vi "Update ceeserver applications.vi"(2 "Source directory":path=path "C:/Users/mw24/Documents/LabVIEW Data/builds") -> (0 "Current file":string)   [LabVIEW 2010]
panel:
  out "uploaded files":string[](array[string])
  out "move to path":path
  out "exe":string[](array[string])
  out "htm":string[](array[string])
  in  "Destination directory":path=path "\\\\ceeserver.cee.cornell.edu\\mw24/Software/Runtime2010"
  out "Current destination":string
  out "file names":string[](array[string])
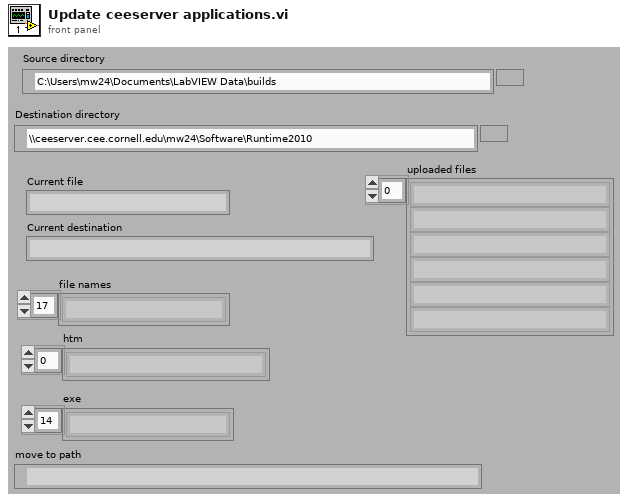
[diagram p1: front panel]
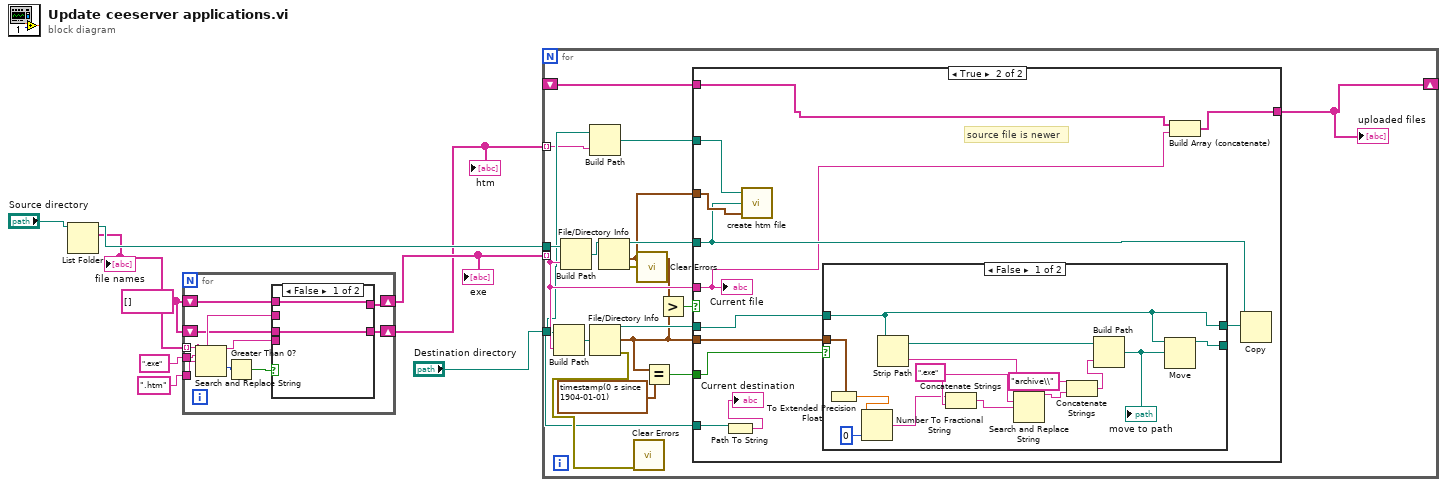
[diagram p0: block diagram]
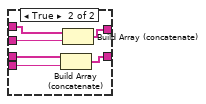
[diagram p2: hidden frame]
diagram:
  w3 = string[] []
  n1 = List Folder(path="Source directory") -> (path out=w8:path, filenames=w6:string[])  [unwired: 3 in, 2 out]
  "file names" <- w6
  n2 = for {
    tunnel: w6 -> [w15] mode=indexing
    tunnel: ".exe" ("search string") -> [w18]
    shift-right: [w17] -> w4
    shift-left: w3 -> [w14]
    shift-right: [w13] -> w2
    shift-left: w3 -> [w11]
    tunnel: ".htm" ("search string") -> [w10]
    n3 = Search and Replace String(input string=w15, search string=w18, replace string=w10) -> (result string=w12:string, offset past replacement=w19:i32)  [unwired: 5 in, 2 out]
    n4 = Greater Than 0?(x=w19) -> (x > 0?=w16:bool)
    n5 = case shown="False" w16 {
      tunnel: [w21 w27] -> w17
      tunnel: w15 -> [_ w26]
      tunnel: w14 -> [w21 w25]
      tunnel: [w20 w24] -> w13
      tunnel: w12 -> [_ w23]
      tunnel: w11 -> [w20 w22]
      frame False {
      }
      frame True {
        n6 = Build Array (concatenate)(w22, w23) -> (w24:string[])
        n7 = Build Array (concatenate)(w25, w26) -> (w27:string[])
      }
    }
  }
  "htm" <- w2
  "exe" <- w4
  n8 = for {
    tunnel: w4 -> [w39] mode=indexing
    tunnel: w8 -> [w45]
    tunnel: "Destination directory" -> [w33]
    tunnel: w2 -> [w32] mode=indexing
    shift-right: [w28] -> _
    shift-left: _ -> [w29]
    n9 = Build Path(base path=w33, name or relative path=w39) -> (appended path=w43:path)
    n10 = Build Path(base path=w45, name or relative path=w39) -> (appended path=w44:path)
    n11 = Build Path(base path=w33, name or relative path=w32) -> (appended path=w31:path)
    n12 = File/Directory Info(path=w43) -> (path out=w41:path, last mod=w30:timestamp, error out=w35:errorcluster)  [unwired: 1 in, 4 out]
    n13 = File/Directory Info(path=w44) -> (path out=w40:path, last mod=w34:timestamp, error out=w38:errorcluster)  [unwired: 1 in, 4 out]
    n14 = call <vilib>:"Clear Errors.vi"("error in (no error)"=w35) -> ()  [unwired: 6 in, 1 out]
    n15 = call <vilib>:"Clear Errors.vi"("error in (no error)"=w38) -> ()  [unwired: 6 in, 1 out]
    n16 = Equal?(x=w30, y=timestamp(0 s since 1904-01-01) ("last mod")) -> (x = y?=w36:bool)
    n17 = Greater?(x=w34, y=w30) -> (0:w42:bool)
    n18 = case shown="True" w42 {
      tunnel: w40 -> [_ w51]
      tunnel: w41 -> [_ w57]
      tunnel: w39 -> [_ w47]
      tunnel: w33 -> [_ w55]
      tunnel: w36 -> [_ w56]
      tunnel: w34 -> [_ w54]
      tunnel: w31 -> [_ w52]
      tunnel: w30 -> [_ w53]
      tunnel: [w46 w48] -> w28
      tunnel: w29 -> [w46 w49]
      frame False {
        # "source file is same age as file on ceeserver"
      }
      frame True {
        # "source file is newer"
        n19 = Path To String(path=w55) -> (string=→"Current destination":string)
        n20 = call "create htm file.vi"("last mod"=w54, "Source path"=w51, "Destination path"=w52) -> ()  [unwired: 2 in]
        n21 = case shown="False" w56 {
          tunnel: w57 -> [w72 w73]
          tunnel: [w72 w73] -> w58
          tunnel: w53 -> [w65 _]
          tunnel: [w69 _] -> _
          frame False {
            w68 = ".exe" ("string")
            n22 = To Extended Precision Float(1:w65) -> (0:w63:ext)
            n23 = Number To Fractional String(number=w63, precision (6)=i16 0) -> (F-format string=w62:string)  [unwired: 2 in]
            n24 = Strip Path(path=w72) -> (stripped path=w70:path, name=w66:string)
            n25 = Concatenate Strings(w62, w68) -> (w67:string)
            n26 = Search and Replace String(input string=w66, search string=w68, replace string=w67) -> (result string=w61:string)  [unwired: 5 in, 3 out]
            n27 = Concatenate Strings("archive\\" ("string"), w61) -> (w60:string)
            n28 = Build Path(base path=w70, name or relative path=w60) -> (appended path=w71:path)
            "move to path" <- w71
            n29 = Move(source path=w72, 10:w71) -> (3:w69:path)  [unwired: 3 in, 2 out]
          }
          frame True {
            # "File doesn't exist"
          }
        }
        n30 = Build Array (concatenate)(w49, w47) -> (w48:string[])
        n31 = Copy(10:w58, 11:w51) -> ()  [unwired: 3 in, 3 out]
        "Current file" <- w47
      }
    }
    "uploaded files" <- w28
  }
